vi "SetResolution.vi"(8 "error in (no error)":errorcluster, 10 "Resolution (hex code)":u8 format="%.0x", 11 "Camera in":refnum<class "Camera.lvclass">) -> (0 "error out":errorcluster, 3 "Camera out":refnum<class "Camera.lvclass">)   [LabVIEW 2020, in "CameraUSB.lvlib" / "Camera.lvclass"]
uses:
  Camera.lvclass
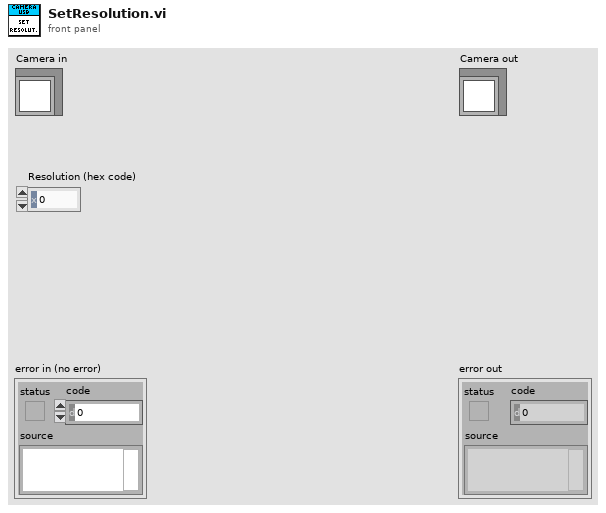
[diagram p1: front panel]
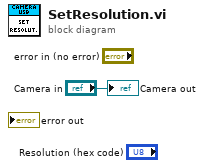
[diagram p0: block diagram]
diagram:
  "Camera out" <- "Camera in"
